vi "Configure Channel (AO).vi"(0 "VISA resource name":refnum<visa-resource-name>, 1 "Channel (0001)":string="0001", 2 "Enable Channel (True)":bool=TRUE, 3 "Type (0: Re-Trans)":u16(ring) items=["Re-Trans", "Manual"], 4 "Range (1: 4-20mA)":u16(ring)=1 items=["0-20mA", "4-20mA"], 5 "Span":T2={"Lower Span (4.000)"=4.0, "Upper Span (20.000)"=20.0} {"Upper Span (20.000)" min=0.0 max=20.0 step=0.001 format="%.3f"; "Lower Span (4.000)" min=0.0 max=20.0 format="%.3g"}, 6 "Reference Channel (When Type is Re-Trans)":T1={"Channel (0001)"="0001", "Kind (0: Input)"=0} {"Kind (0: Input)" items=["Input", "Math", "Com"]}, 7 "error in":errorcluster, 9 "Preset Value (0.000)":dbl min=0.0 max=22.0 format="%.3f") -> (20 "VISA resource name out":refnum<visa-resource-name>, 21 "Channel":string, 27 "error out":errorcluster)   [LabVIEW 2020, in "Yokogawa GX Series.lvlib"]
doc: "Sets the AO range.\n\nCommand: SRangeAO"
uses:
  <instrlib>/Yokogawa GX Series/Yokogawa GX Series.lvlib
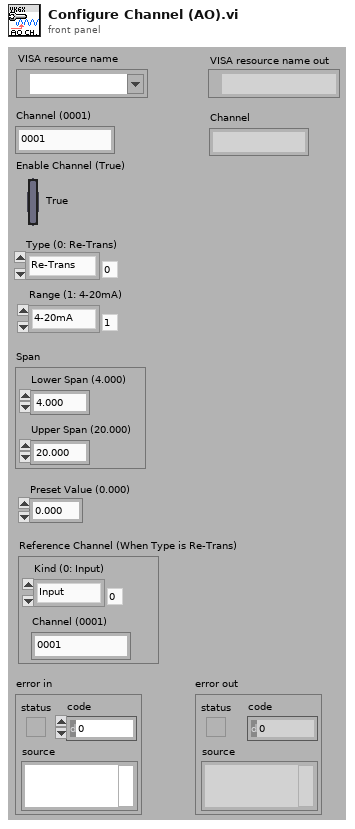
[diagram p1: front panel]
types:
  T1 = cluster{"Channel (0001)":string, "Kind (0: Input)":u16}
  T2 = cluster{"Lower Span (4.000)":dbl, "Upper Span (20.000)":dbl}
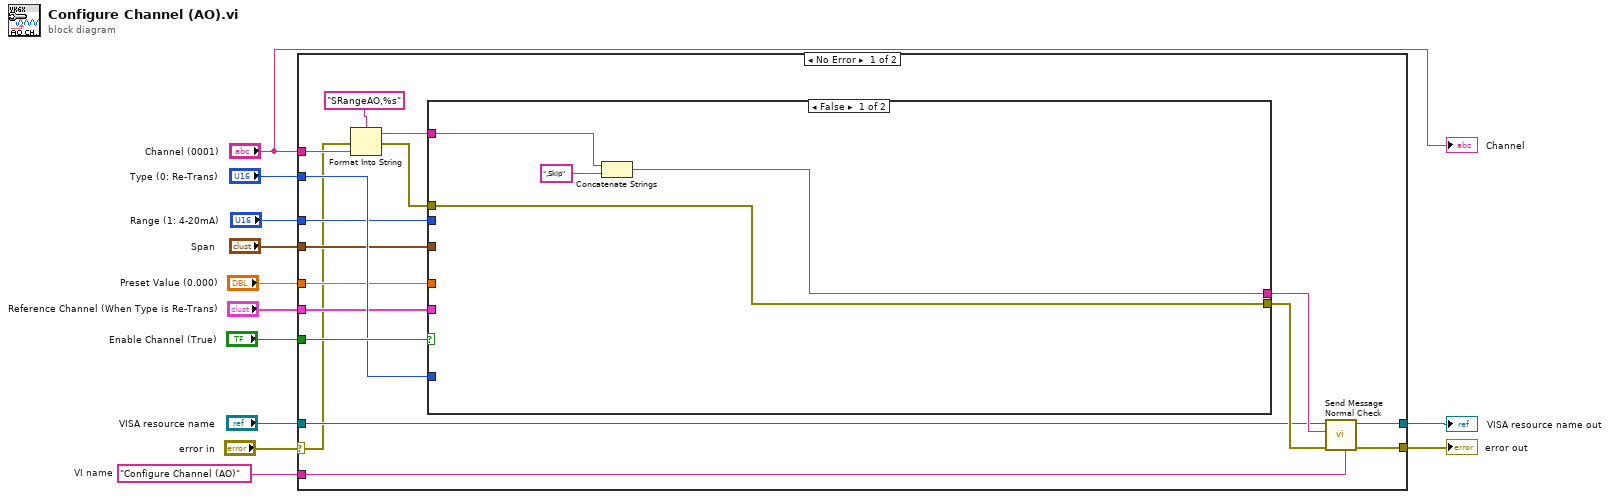
[diagram p0: block diagram]
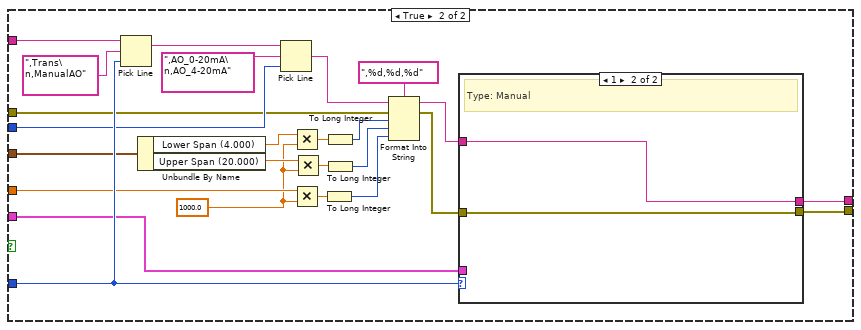
[diagram p2: hidden frame]
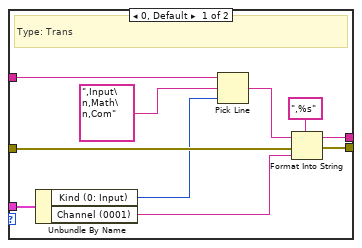
[diagram p3: hidden frame]
diagram:
  w12 = "Configure Channel (AO)"  # VI name
  n1 = case shown="No Error" "error in" {
    selector: "error in" -> [w13 w72]
    tunnel: [w26 w71] -> w4
    tunnel: [w25 w72] -> w1
    tunnel: w12 -> [w22 _]
    tunnel: "Channel (0001)" -> [w21 _]
    tunnel: "Enable Channel (True)" -> [w20 _]
    tunnel: "Type (0: Re-Trans)" -> [w19 _]
    tunnel: "Range (1: 4-20mA)" -> [w18 _]
    tunnel: "Span" -> [w17 _]
    tunnel: "Preset Value (0.000)" -> [w16 _]
    tunnel: "Reference Channel (When Type is Re-Trans)" -> [w15 _]
    tunnel: "VISA resource name" -> [w14 w71]
    frame No Error {
      n2 = Format Into String(format string="SRangeAO,%s", error in=w13, w21) -> (resulting string=w27:string, error out=w28:errorcluster)  [unwired: 1 in]
      n3 = case shown="False" w20 {
        tunnel: w28 -> [w30 w51]
        tunnel: [w30 w42] -> w24
        tunnel: w27 -> [w31 w58]
        tunnel: [w32 w34] -> w23
        tunnel: w19 -> [_ w56]
        tunnel: w18 -> [_ w53]
        tunnel: w17 -> [_ w50]
        tunnel: w16 -> [_ w48]
        tunnel: w15 -> [_ w45]
        frame False {
          n4 = Concatenate Strings(w31, ",Skip") -> (w32:string)
        }
        frame True {
          w38 = 1000.0
          n5 = Pick Line(string ("")=w58, multi-line string=",Trans\n,ManualAO", line index=w56) -> (output string=w55:string)
          n6 = Unbundle By Name(w50) -> ("Lower Span (4.000)"=w40:dbl, "Upper Span (20.000)"=w39:dbl)
          n7 = Pick Line(string ("")=w55, multi-line string=",AO_0-20mA\n,AO_4-20mA", line index=w53) -> (output string=w52:string)
          n8 = Multiply(x=w40, y=w38) -> (x*y=w37:dbl)
          n9 = Multiply(x=w48, y=w38) -> (x*y=w47:dbl)
          n10 = Multiply(x=w39, y=w38) -> (x*y=w36:dbl)
          n11 = To Long Integer(number=w47) -> (32bit integer=w46:i32)
          n12 = To Long Integer(number=w37) -> (32bit integer=w35:i32)
          n13 = To Long Integer(number=w36) -> (32bit integer=w41:i32)
          n14 = Format Into String(format string=",%d,%d,%d", initial string=w52, error in=w51, w35, w41, w46) -> (resulting string=w43:string, error out=w44:errorcluster)
          n15 = case shown="1" w56 {
            tunnel: w45 -> [w68 _]
            tunnel: w44 -> [w67 w69]
            tunnel: w43 -> [w64 w70]
            tunnel: [w60 w69] -> w42
            tunnel: [w59 w70] -> w34
            frame 0, Default {
              # "Type: Trans"
              n16 = Unbundle By Name(w68) -> ("Kind (0: Input)"=w62:u16, "Channel (0001)"=w65:string)
              n17 = Pick Line(string ("")=w64, multi-line string=",Input\n,Math\n,Com", line index=w62) -> (output string=w61:string)
              n18 = Format Into String(format string=",%s", initial string=w61, error in=w67, w65) -> (resulting string=w59:string, error out=w60:errorcluster)
            }
            frame 1 {
              # "Type: Manual"
            }
          }
        }
      }
      n19 = call <instrlib>:"Send Message Normal Check.vi"("Source (\"\")"=w22, "error in (no error)"=w24, "Send Message (\"\")"=w23, "VISA resource name"=w14) -> ("error out"=w25:errorcluster, "VISA resource name out"=w26:refnum<visa-resource-name>)  [unwired: 2 in, 4 out]
    }
    frame Error {
    }
  }
  "VISA resource name out" <- w4
  "error out" <- w1
  "Channel" <- "Channel (0001)"
